vi "Datasheet Create HTM.vi"(8 "error in (no error)":errorcluster, 9 "sxTemplateId":string, 10 "template":string, 11 "array out":T1) -> (0 "error out":errorcluster, 3 "report":path)   [LabVIEW 2011]
uses:
  Addons/internet/utils/keyedarr.llb/Keyed Array.ctl
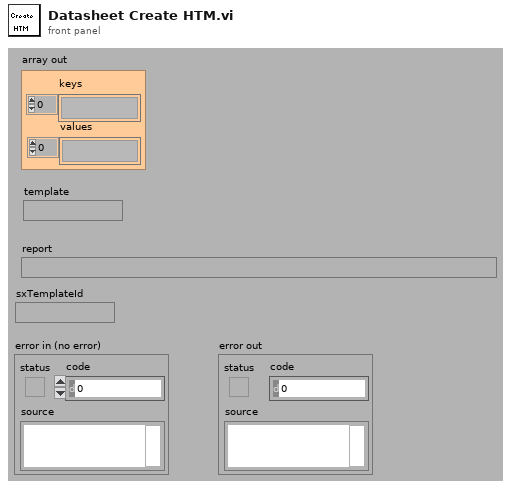
[diagram p1: front panel]
types:
  T1 = typedef "Keyed Array.ctl" = cluster{"keys":string[], "values":string[]}
  T2 = enum16{"open", "replace", "create", "open or create", "replace or create", "replace or create with confirmation"}
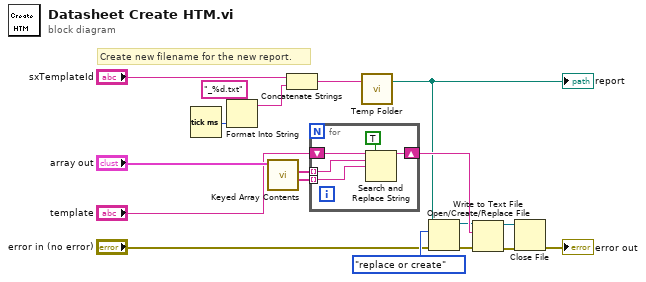
[diagram p0: block diagram]
diagram:
  # "Create new filename for the new report."
  n1 = Tick Count (ms)() -> (millisecond timer value=w6:u32)
  n2 = Format Into String(format string="_%d.txt", w6) -> (resulting string=w5:string)  [unwired: 2 in, 1 out]
  n3 = call "Keyed Array Contents.vi"("array in"="array out") -> ("values"=w15:string[], "keys"=w14:string[])  [unwired: 5 out]
  n4 = Concatenate Strings("sxTemplateId", w5) -> (w3:string)
  n5 = for {
    shift-right: [w21] -> w16
    shift-left: "template" -> [w22]
    tunnel: w14 -> [w20] mode=indexing
    tunnel: w15 -> [w19] mode=indexing
    n6 = Search and Replace String(replace all?=TRUE, input string=w22, search string=w20, replace string=w19) -> (result string=w21:string)  [unwired: 1 in, 6 out]
  }
  n7 = call "Temp Folder.vi"("Relative Path (\"\")"=w3) -> ("Temp Folder"=w2:path)  [unwired: 2 in]
  "report" <- w2
  n8 = Open/Create/Replace File(file path (use dialog)=w2, error in="error in (no error)", operation (0:open)=T2."replace or create") -> (refnum out=w9:refnum<file>, error out=w10:errorcluster)  [unwired: 4 out]
  n9 = Write to Text File(file (use dialog)=w9, text=w16, error in=w10) -> (refnum out=w11:refnum<file>, error out=w12:errorcluster)  [unwired: 2 out]
  n10 = Close File(refnum=w11, error in=w12) -> (error out=→"error out":errorcluster)  [unwired: 1 out]
